vi "Create TrafficMap.vi"(5 "TrafficMap in":refnum<class "TrafficMap.lvclass">, 8 "error in (no error)":errorcluster, 11 "Zones":string[](array[string])) -> (0 "error out":errorcluster, 3 "TrafficMap":refnum<class "TrafficMap.lvclass">)   [LabVIEW 2017, in "TrafficMap.lvclass"]
uses:
  TrafficMap.lvclass
  TrafficMap.lvclass/TrafficMap.ctl
  Zone/Zone.lvclass
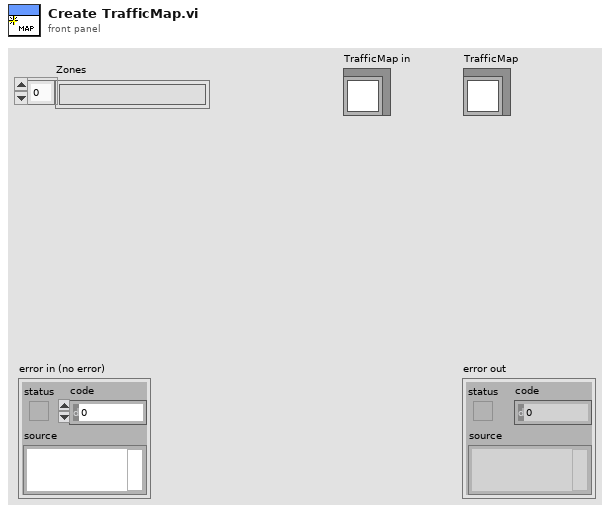
[diagram p1: front panel]
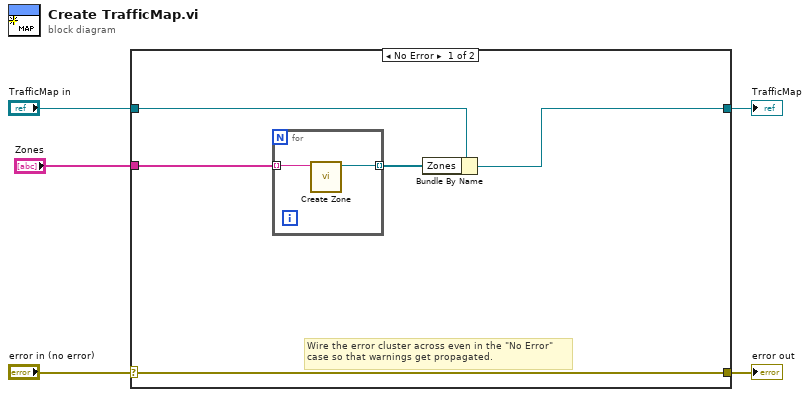
[diagram p0: block diagram]
diagram:
  n1 = case shown="No Error" "error in (no error)" {
    selector: "error in (no error)" -> [w10 w14]
    tunnel: [w10 w14] -> w4
    tunnel: [w6 w13] -> w2
    tunnel: "TrafficMap in" -> [w7 w13]
    tunnel: "Zones" -> [w8 _]
    frame No Error {
      # "Wire the error cluster across even in the \"No Error\"\ncase so that warnings get propagated."
      n2 = for {
        tunnel: [w12] -> w9 mode=indexing
        tunnel: w8 -> [w11] mode=indexing
        n3 = call "Create Zone.vi"("Zone Name"=w11) -> ("Zone out"=w12:refnum<class "Zone.lvclass">)  [unwired: 9 in, 1 out]
      }
      n4 = Bundle By Name(cluster=w7, "Zones"=w9) -> (w6:refnum<class "TrafficMap.lvclass">)
    }
    frame Error {
    }
  }
  "error out" <- w4
  "TrafficMap" <- w2
